vi "hwOperation_hwConnect.vi"(7 "hwType":string="Simulation", 8 "error in (no error)":errorcluster) -> (0 "error out":errorcluster, 2 "Connect?":bool, 3 "hwDriverRef":T1)   [LabVIEW 2016]
uses:
  QX/hw_QX_hwDriverRef.ctl
  C:/Users/CL/Desktop/ZcDAQprj0811/ZcDAQprj/Modules/DAQ-Device/Hardware Drivers/QX/HBM LabVIEW Driver/DLLs/Hbm.Api.Common.dll
  QX/HBM LabVIEW Driver/DLLs/Hbm.Api.Common.dll
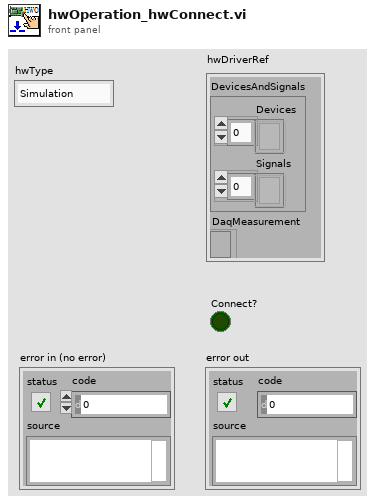
[diagram p1: front panel]
types:
  T1 = typedef "hw_QX_hwDriverRef.ctl" = cluster{"DevicesAndSignals":cluster{"Devices":refnum<k24>[], "Signals":refnum<k24>[]}, "DaqMeasurement":refnum<k24>}
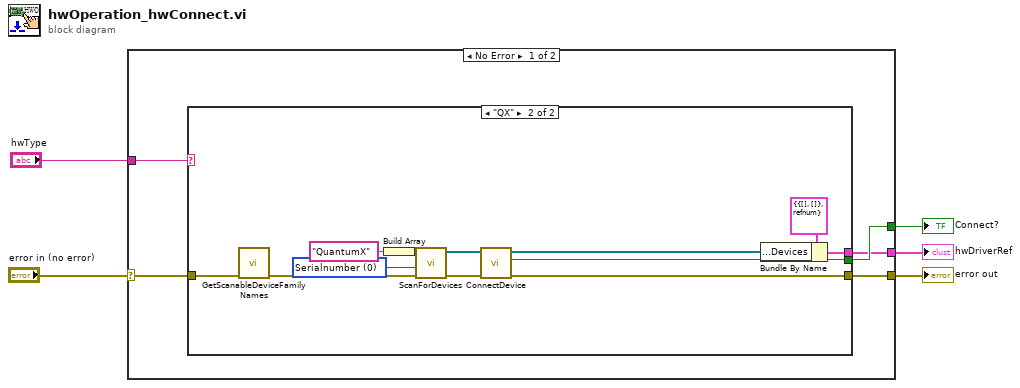
[diagram p0: block diagram]
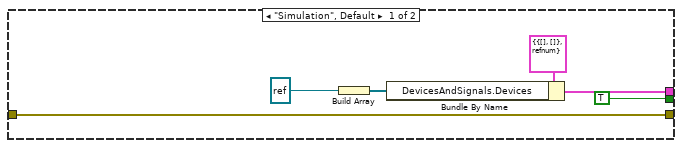
[diagram p2: hidden frame]
diagram:
  n1 = case shown="No Error" "error in (no error)" {
    selector: "error in (no error)" -> [w9 w29]
    tunnel: [w10 w29] -> w5
    tunnel: "hwType" -> [w8 _]
    tunnel: [w7 _] -> w2
    tunnel: [w6 _] -> w1
    frame No Error {
      n2 = case shown="\"QX\"" w8 {
        tunnel: [w16 w27] -> w10
        tunnel: w9 -> [w16 w21]
        tunnel: [TRUE ("Result") w20] -> w7
        tunnel: [w11 w17] -> w6
        frame "Simulation", Default {
          n3 = Build Array(refnum<k24> refnum (".NET Refnum")) -> (w12:refnum<k24>[])
          n4 = Bundle By Name(cluster=T1 {"DevicesAndSignals"={"Devices"=[], "Signals"=[]}, "DaqMeasurement"=refnum} ("hwDriverRef"), "DevicesAndSignals.Devices"=w12) -> (w11:T1)
        }
        frame "QX" {
          w23 = 0 items=["Serialnumber", "Name", "IpAddress"] ("SortedBy")
          n5 = call "GetScanableDeviceFamilyNames.vi"("Error in"=w21) -> ("Error out"=w24:errorcluster)  [unwired: 8 in, 2 out]
          n6 = Build Array("QuantumX") -> (w22:string[])
          n7 = call "ScanForDevices.vi"("Error in"=w24, "SortedBy"=w23, "AvailableDeviceFamilies"=w22) -> ("Error out"=w26:errorcluster, "Devices"=w28:refnum<k24>[])  [unwired: 7 in]
          n8 = call "ConnectDevice.vi"("Error in"=w26, "Devices"=w28) -> ("Error out"=w27:errorcluster, "Result"=w20:bool, "Devices"=w18:refnum<k24>[])  [unwired: 7 in]
          n9 = Bundle By Name(cluster=T1 {"DevicesAndSignals"={"Devices"=[], "Signals"=[]}, "DaqMeasurement"=refnum} ("hwDriverRef"), "DevicesAndSignals.Devices"=w18) -> (w17:T1)
        }
      }
    }
    frame Error {
    }
  }
  "error out" <- w5
  "Connect?" <- w2
  "hwDriverRef" <- w1
